vi "Highlight Data Accessor.vi"(7 "Full Element Name":string[](array[string]), 8 "error in (no error)":errorcluster, 10 "Cluster":T1, 11 "JKI SM in":refnum<class "JKI SM.lvclass">) -> (0 "error out":errorcluster, 3 "JKI SM out":refnum<class "JKI SM.lvclass">)   [LabVIEW 2013]
uses:
  JKI State Machine API/source/JKI SM/JKI SM.lvclass
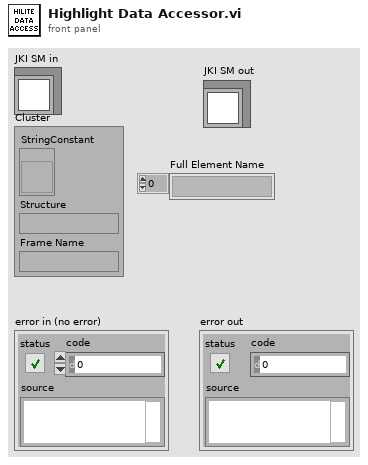
[diagram p1: front panel]
types:
  T1 = cluster{"StringConstant":refnum<vi>, "Structure":string, "Frame Name":string}
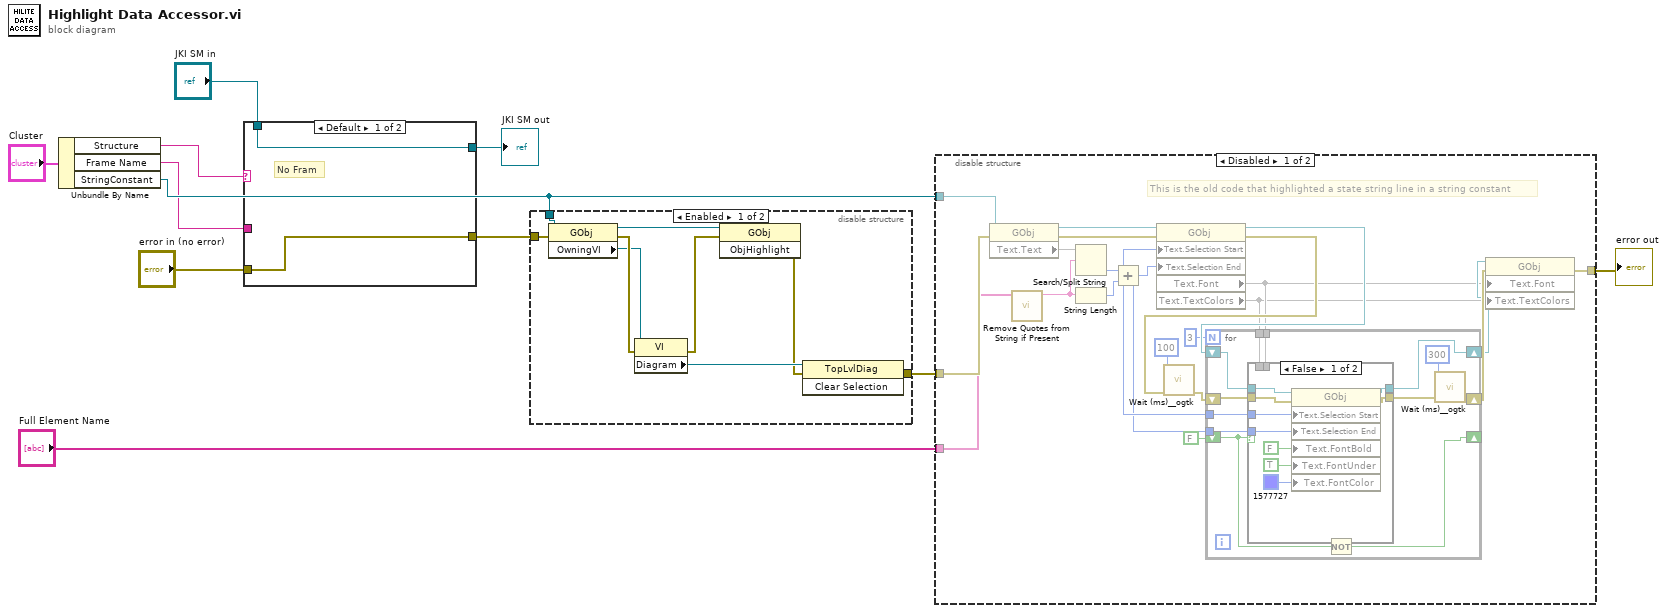
[diagram p0: block diagram]
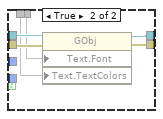
[diagram p2: hidden frame]
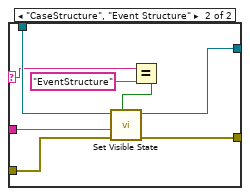
[diagram p4: hidden frame]
diagram:
  n1 = Unbundle By Name("Cluster") -> ("Structure"=w1:string, "Frame Name"=w2:string, "StringConstant"=w3:refnum<vi>)
  n2 = case shown="Default" w1 {
    selector: w1 -> [_ w15]
    tunnel: [w12 w21] -> w11
    tunnel: "error in (no error)" -> [w12 w20]
    tunnel: "JKI SM in" -> [w13 w19]
    tunnel: [w13 w18] -> w7
    tunnel: w2 -> [_ w17]
    frame Default {
      # "No Fram"
    }
    frame "CaseStructure", "Event Structure" {
      n3 = Equal?(x=w15, y="EventStructure") -> (x = y?=w14:bool)
      n4 = call "Set Visible State.vi"("Event Structure (F: Case Structure)"=w14, "error in (no error)"=w20, "State Name"=w17, "JKI SM in"=w19) -> ("error out"=w21:errorcluster, "JKI SM out"=w18:refnum<class "JKI SM.lvclass">)  [unwired: 6 in]
    }
  }
  "JKI SM out" <- w7
  n5 = disable-structure shown="Enabled" {
    disable-tunnel: w11 -> [w27 w31]
    disable-tunnel: [w25 w31] -> w6
    disable-tunnel: w3 -> [w22 _]
    frame Enabled {
      n6 = property class="GObj"(reference=w22, error in=w27) -> (reference out=w23:refnum<vi>, error out=w28:errorcluster, "OwningVI"=w26:refnum<vi>)
      n7 = property class="VI"(reference=w26, error in=w28) -> (error out=w29:errorcluster, "Diagram"=w30:refnum<vi>)  [unwired: 1 out]
      n8 = invoke class="GObj" method="ObjHighlight"(reference=w23, error in=w29) -> (error out=w24:errorcluster)  [unwired: 1 in, 2 out]
      n9 = invoke class="TopLvlDiag" method="Clear Selection"(reference=w30, error in=w24) -> (error out=w25:errorcluster)  [unwired: 1 in, 2 out]
    }
    frame Disabled {
    }
  }
  n10 = disable-structure shown="Disabled" {
    disable-tunnel: w6 -> [w49 w80]
    disable-tunnel: "Full Element Name" -> [w46 _]
    disable-tunnel: [w43 w80] -> w4
    disable-tunnel: w3 -> [w35 _]
    frame Disabled {
      # "This is the old code that highlighted a state string line in a string constant"
      n11 = property class="GObj"(reference=w35, error in=w49) -> (reference out=w51:refnum<vi>, error out=w48:errorcluster, "Text.Text"=w52)
      n12 = call "Remove Quotes from String if Present.vi"("String"=w46) -> ("String with Quotes Removed"=w47:string)  [unwired: 10 in]
      n13 = Search/Split String(string=w52, search string/char (-)=w47) -> (offset of match=w33:i32)  [unwired: 1 in, 2 out]
      n14 = String Length(string=w47) -> (length=w50:i32)
      n15 = Add(x=w33, y=w50) -> (x+y=w32:i32)
      n16 = property class="GObj"(reference=w51, error in=w48, "Text.Selection Start"=w33, "Text.Selection End"=w32) -> (reference out=w45:refnum<vi>, error out=w39:errorcluster, "Text.Font"=w36, "Text.TextColors"=w34)
      n17 = call <userlib>:"Wait (ms)__ogtk.vi"("error in (no error)"=w39, "milliseconds to wait"=u32 100) -> ("error out"=w40:errorcluster)  [unwired: 8 in, 1 out]
      n18 = for {
        N: 3 -> [_]
        shift-right: [w61] -> w44
        shift-left: w40 -> [w59]
        shift-right: [w60] -> w42
        shift-left: w45 -> [w64]
        shift-right: [w57] -> _
        shift-left: FALSE -> [w58]
        tunnel: w36 -> [w56]
        tunnel: w34 -> [w55]
        tunnel: w33 -> [w54]
        tunnel: w32 -> [w53]
        n19 = case shown="False" w58 {
          tunnel: w64 -> [w73 w79]
          tunnel: [w72 w77] -> w63
          tunnel: [w71 w78] -> w60
          tunnel: w59 -> [w68 w76]
          tunnel: w56 -> [_ w75]
          tunnel: w55 -> [_ w74]
          tunnel: w54 -> [w66 _]
          tunnel: w53 -> [w65 _]
          frame False {
            n20 = property class="GObj"(reference=w73, error in=w68, "Text.Selection Start"=w66, "Text.Selection End"=w65, "Text.FontBold"=FALSE ("Text.Font:Bold"), "Text.FontUnder"=TRUE ("Text.Font:Bold"), "Text.FontColor"=u32 1577727) -> (reference out=w71:refnum<vi>, error out=w72:errorcluster)
          }
          frame True {
            n21 = property class="GObj"(reference=w79, error in=w76, "Text.Font"=w75, "Text.TextColors"=w74) -> (reference out=w78:refnum<vi>, error out=w77:errorcluster)
          }
        }
        n22 = Not(x=w58) -> (.not. x?=w57:bool)
        n23 = call <userlib>:"Wait (ms)__ogtk.vi"("error in (no error)"=w63, "milliseconds to wait"=u32 300) -> ("error out"=w61:errorcluster)  [unwired: 8 in, 1 out]
      }
      n24 = property class="GObj"(reference=w42, error in=w44, "Text.Font"=w36, "Text.TextColors"=w34) -> (error out=w43:errorcluster)  [unwired: 1 out]
    }
    frame Enabled {
    }
  }
  "error out" <- w4
